vi "variantTypeToX.vi"   [LabVIEW 2011]
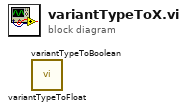
[diagram p0: block diagram]
diagram:
  n1 = call "variantTypeToFloat.vi"() -> ()  [unwired: 12 in]
  n2 = call "variantTypeToBoolean.vi"() -> ()  [unwired: 10 in, 2 out]
